vi "Esercitazione 7 - Moto Proiettile.vi"() -> ()   [LabVIEW 2018]
panel:
  in  "Altezza obbiettivo":i32
  in  "Posizione obiettivo":dbl=500.0 format="%#_13g"
  in  "Distanza barriera":dbl=500.0 format="%#_13g"
  in  "Altezza barriera":i32=20
  in  "y0":dbl
  out "XY Graph":cluster{dbl[], dbl[]}[](graph)
  in  "V0":dbl
  in  "Angolo":dbl
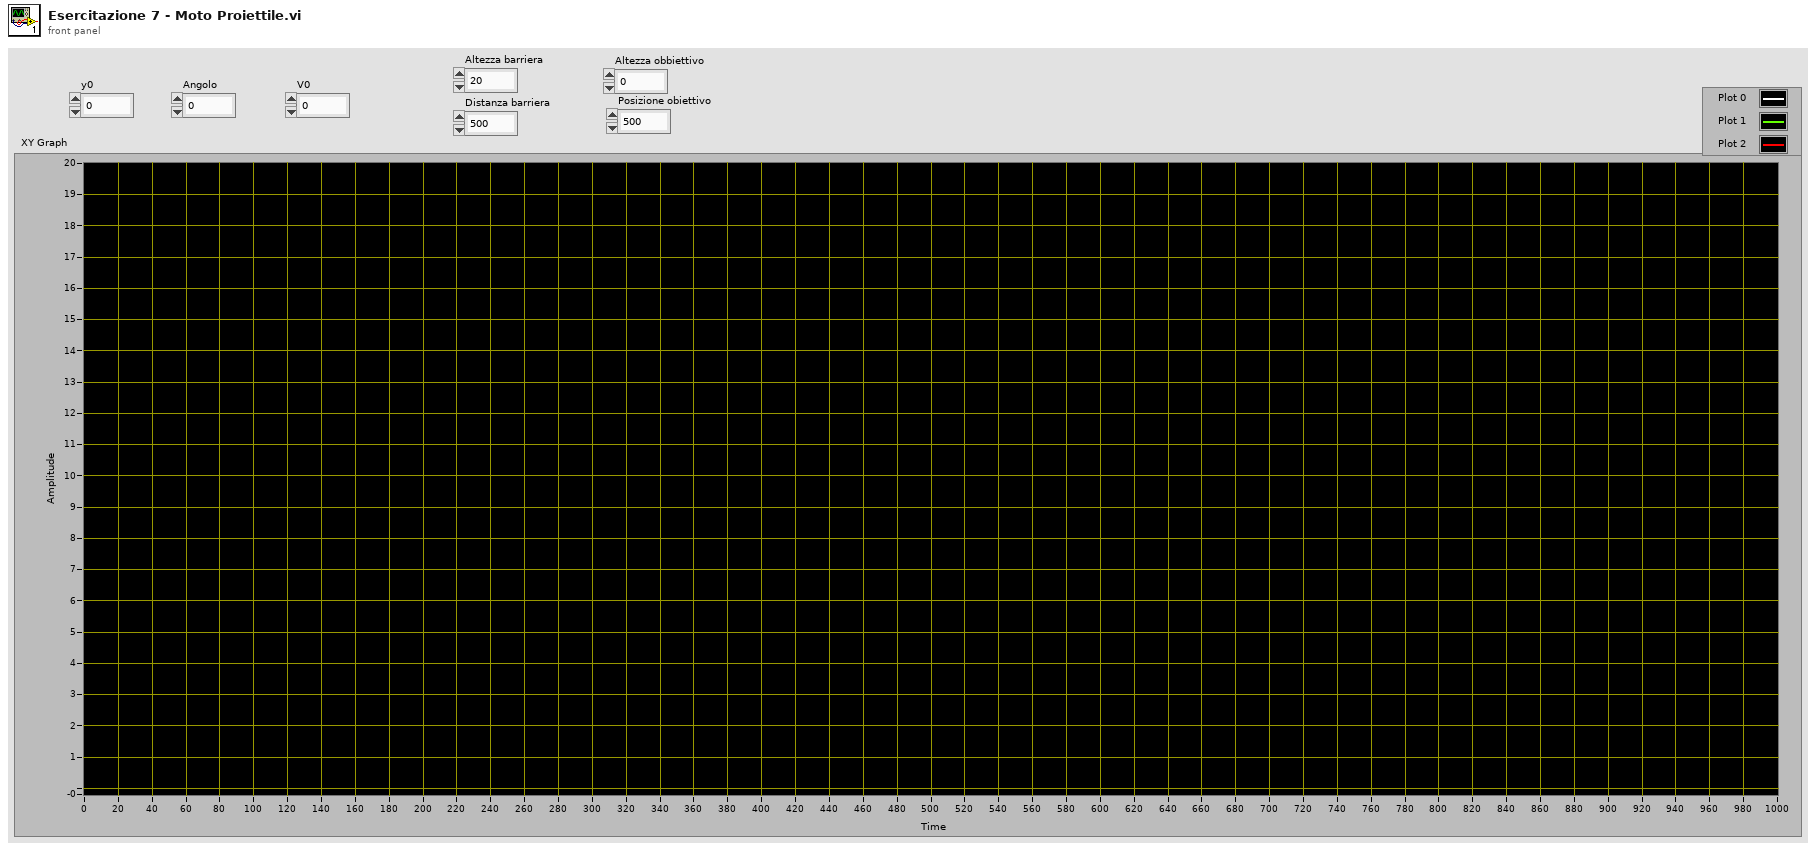
[diagram p1: front panel]
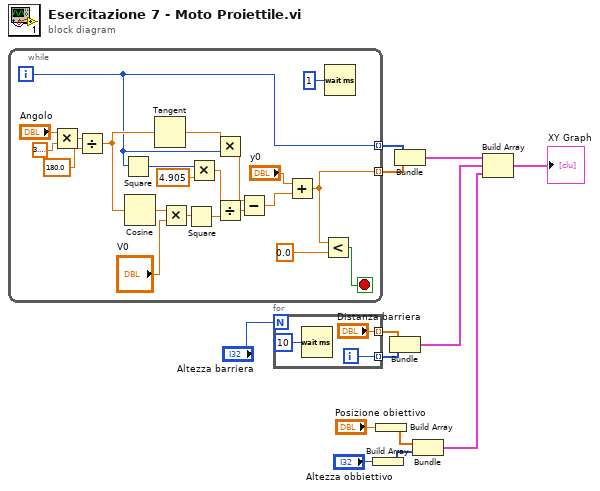
[diagram p0: block diagram]
diagram:
  n1 = while {
    tunnel: [w14] -> w10 mode=indexing
    tunnel: [w15] -> w9 mode=indexing
    i -> [w14]
    stop <- w24 stop-if-true
    n2 = Multiply(x="Angolo", y=3.141592653589793) -> (x*y=w21:dbl)
    n3 = Divide(x=w21, y=180.0) -> (x/y=w20:dbl)
    n4 = Square(x=w14) -> (x^2=w26:i32)
    n5 = Cosine(x=w20) -> (cos(x)=w33:dbl)
    n6 = Tangent(1:w20) -> (0:w35:dbl)
    n7 = Multiply(x=w33, y="V0") -> (x*y=w31:dbl)
    n8 = Square(x=w31) -> (x^2=w30:dbl)
    n9 = Multiply(x=w26, y=4.905) -> (x*y=w28:dbl)
    n10 = Multiply(x=w35, y=w14) -> (x*y=w34:dbl)
    n11 = Divide(x=w28, y=w30) -> (x/y=w29:dbl)
    n12 = Subtract(x=w34, y=w29) -> (x-y=w17:dbl)
    n13 = Add(x="y0", y=w17) -> (x+y=w15:dbl)
    n14 = Less?(x=w15, y=0.0) -> (x < y?=w24:bool)
    n15 = Wait (ms)(milliseconds to wait=u32 1) -> ()  [unwired: 1 out]
  }
  n16 = for {
    N: "Altezza barriera" -> [_]
    tunnel: ["Distanza barriera"] -> w13 mode=indexing
    tunnel: [w37] -> w12 mode=indexing
    i -> [w37]
    n17 = Wait (ms)(milliseconds to wait=u32 10) -> ()  [unwired: 1 out]
  }
  n18 = Build Array("Altezza obbiettivo") -> (w1:i32[])
  n19 = Build Array("Posizione obiettivo") -> (w3:dbl[])
  n20 = Bundle(w13, w12) -> (w7:cluster{dbl[], i32[]})  [unwired: 1 in]
  n21 = Bundle(w10, w9) -> (w8:cluster{i32[], dbl[]})  [unwired: 1 in]
  n22 = Bundle(w3, w1) -> (w5:cluster{dbl[], i32[]})  [unwired: 1 in]
  n23 = Build Array(w8, w7, w5) -> (→"XY Graph":cluster{dbl[], dbl[]}[])
